vi "Launch Root UIA.vi"(8 "error in (no error)":errorcluster, 10 "Actor Name":string, 11 "UI_Actor in":refnum<class "UI_Actor.lvclass">) -> (0 "error out":errorcluster, 3 "Actor's Enqueuer":refnum<class "Message Enqueuer.lvclass">)   [LabVIEW 2020, in "UI_Actor.lvlib" / "UI_Actor.lvclass"]
doc: "Lance l'actor root -> C'est la supervision.\nActor Name est facultatif, et en accès lecture via les propriétés.\n\n<b> ATTENTION </b> Ce VI affecte le AppPath. Une hierarchie de dossier est à respecter à la lettre.\nIl faut <b> impérativement </b> que les choses soient organisées comme suit:\n - Dossier de l'application\n - Launch App .vi (vi qui lance l'acteur root)\n - Acteur Root (dossier de l'acteur root, automatiquement créé par le wizard NI)"
uses:
  UI_Actor.lvclass
  D:/Projets/STEP AT/UI Actor/support/Actor Framework.lvlibp/1abvi3w/vi.lib/ActorFramework/Actor/Actor.lvclass
  support/Actor Framework.lvlibp/1abvi3w/vi.lib/ActorFramework/Message Enqueuer/Message Enqueuer.lvclass
  UI_Actor.lvclass/UI_Actor.ctl
  support/Actor Framework.lvlibp/1abvi3w/vi.lib/ActorFramework/Actor/Actor.lvclass
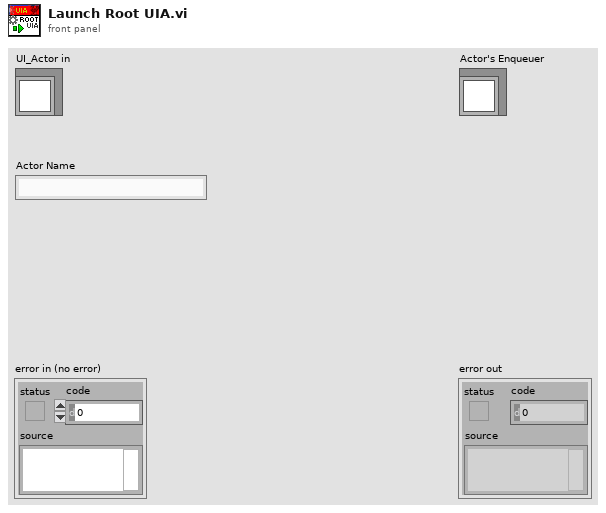
[diagram p1: front panel]
types:
  T1 = enum32{"invalid app kind", "Development System", "Run Time System", "Student Edition", "Embedded LabVIEW", "Evaluation", "Custom"}
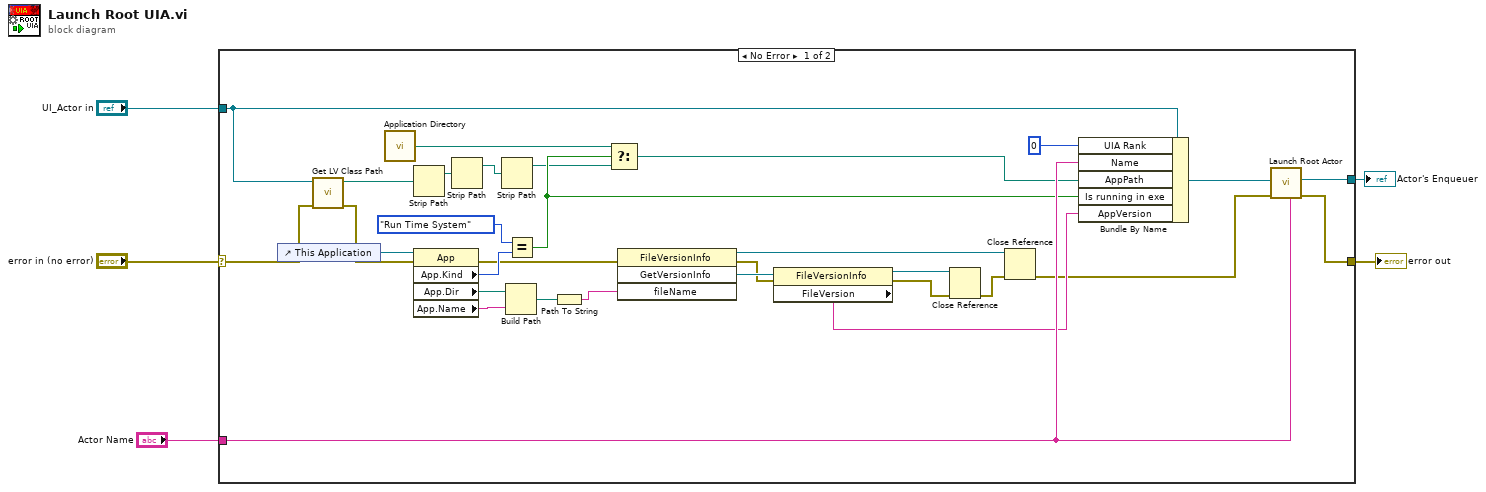
[diagram p0: block diagram]
diagram:
  n1 = case shown="No Error" "error in (no error)" {
    selector: "error in (no error)" -> [w7 w37]
    tunnel: [w35 w37] -> w4
    tunnel: "UI_Actor in" -> [w25 _]
    tunnel: [w36 _] -> w2
    tunnel: "Actor Name" -> [w33 _]
    frame No Error {
      n2 = control-ref of="This Application"() -> (w29:refnum<vi>)
      n3 = call <vilib>:"Get LV Class Path.vi"("error in (no error)"=w7, "object"=w25) -> ("error out"=w6:errorcluster, "class path"=w22:path)  [unwired: 8 in]
      n4 = call <vilib>:"Application Directory.vi"() -> ("Application Directory"=w32:path)
      n5 = Strip Path(path=w22) -> (stripped path=w26:path)  [unwired: 1 out]
      n6 = property class="App"(reference=w29, error in=w6) -> (error out=w11:errorcluster, "App.Kind"=w30:T1, "App.Dir"=w13:path, "App.Name"=w12:string)  [unwired: 1 out]
      n7 = Strip Path(path=w26) -> (stripped path=w24:path)  [unwired: 1 out]
      n8 = Strip Path(path=w24) -> (stripped path=w23:path)  [unwired: 1 out]
      n9 = Build Path(base path=w13, name or relative path=w12) -> (appended path=w14:path)
      n10 = Equal?(x=T1."Run Time System" ("y"), y=w30) -> (x = y?=w27:bool)
      n11 = Path To String(path=w14) -> (string=w19:string)
      n12 = Select(t=w32, s=w27, f=w23) -> (s? t:f=w28:path)
      n13 = invoke class="FileVersionInfo" method="GetVersionInfo"(error in=w11, "fileName"=w19) -> (reference out=w15:refnum<k24>, error out=w20:errorcluster, "GetVersionInfo"=w21:refnum<k24>)  [unwired: 2 in, 1 out]
      n14 = property class="FileVersionInfo"(reference=w21, error in=w20) -> (reference out=w18:refnum<k24>, error out=w17:errorcluster, "FileVersion"=w10:string)
      n15 = Close Reference(reference=w18, error in (no error)=w17) -> (error out=w16:errorcluster)
      n16 = Close Reference(reference=w15, error in (no error)=w16) -> (error out=w9:errorcluster)
      n17 = Bundle By Name(cluster=w25, "UIA Rank"=0, "Name"=w33, "AppPath"=w28, "Is running in exe"=w27, "AppVersion"=w10) -> (w8:refnum<class "UI_Actor.lvclass">)
      n18 = call "Launch Root Actor.vi"("Debug Alias"=w33, "error in (no error)"=w9, "Actor"=w8) -> ("error out"=w35:errorcluster, "Actor's Enqueuer"=w36:refnum<class "Message Enqueuer.lvclass">)  [unwired: 7 in]
    }
    frame Error {
    }
  }
  "error out" <- w4
  "Actor's Enqueuer" <- w2
